vi "_25_Sample_qsns_9[1].vi"() -> ()   [LabVIEW 2020]
panel:
  out "all upper case string":string
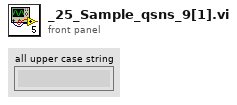
[diagram p1: front panel]
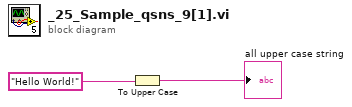
[diagram p0: block diagram]
diagram:
  n1 = To Upper Case(1:"Hello World!") -> (0:→"all upper case string":string)
